vi "startup.vi"(8 "error in (no error)":errorcluster, 11 "PixelflySettings in":refnum<class "PixelflySettings.lvclass">) -> (0 "error out":errorcluster, 3 "PixelflySettings out":refnum<class "PixelflySettings.lvclass">)   [LabVIEW 2009, in "Tools.lvlib" / "Settings.lvlib" / "PixelflySettings.lvclass"]
uses:
  PixelflySettings.lvclass
  Filing/FileSystem/FileSystem.lvclass
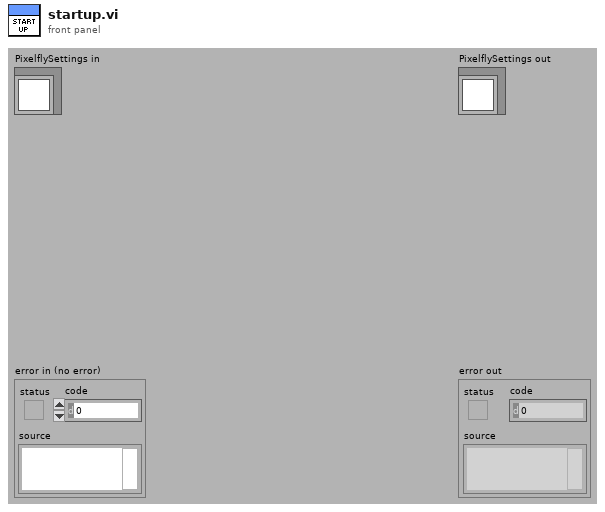
[diagram p1: front panel]
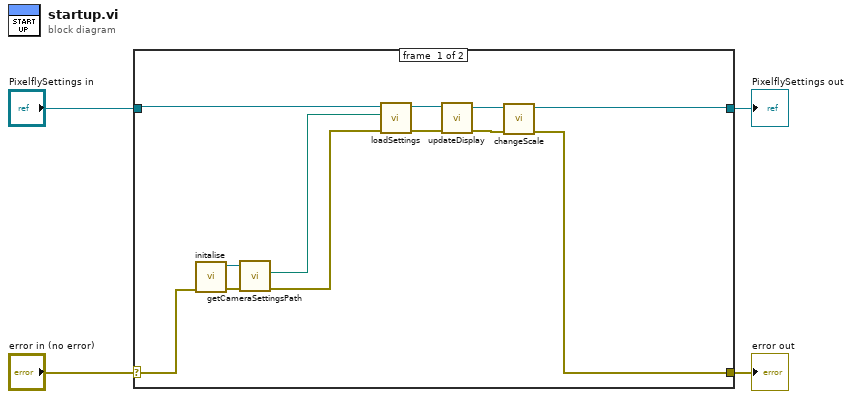
[diagram p0: block diagram]
diagram:
  n1 = case shown="No Error" "error in (no error)" {
    selector: "error in (no error)" -> [w10 w18]
    tunnel: [w5 w18] -> w3
    tunnel: [w6 w17] -> w1
    tunnel: "PixelflySettings in" -> [w16 w17]
    frame #0 {
      n2 = call "initalise.vi"("error in (no error)"=w10) -> ("error out"=w12:errorcluster, "FileSystem out"=w13:refnum<class "FileSystem.lvclass">)  [unwired: 9 in]
      n3 = call-dynamic "getCameraSettingsPath.vi"("error in (no error)"=w12, "FileSystem.lvclass in"=w13) -> ("error out"=w9:errorcluster, "CameraSettingsPath"=w11:path)  [unwired: 7 in, 1 out]
      n4 = call-dynamic "loadSettings.vi"("error in (no error)"=w9, "Path"=w11, "PixelflySettings in"=w16) -> ("error out"=w14:errorcluster, "PixelflySettings out"=w15:refnum<class "PixelflySettings.lvclass">)  [unwired: 7 in]
      n5 = call "updateDisplay.vi"("error in (no error)"=w14, "PixelflySettings in"=w15) -> ("error out"=w7:errorcluster, "PixelflySettings out"=w8:refnum<class "PixelflySettings.lvclass">)  [unwired: 8 in]
      n6 = call "changeScale.vi"("error in (no error)"=w7, "PixelflySettings in"=w8) -> ("error out"=w5:errorcluster, "PixelflySettings out"=w6:refnum<class "PixelflySettings.lvclass">)  [unwired: 8 in]
    }
    frame #1 {
    }
  }
  "error out" <- w3
  "PixelflySettings out" <- w1
